vi "parseReadCalibrationResponse.vi"(8 "error in (no error)":errorcluster, 10 "DynamicFrameParser":refnum<class "DynamicFrameParser.lvclass">, 11 "ILC in":refnum<class "ILC.lvclass">) -> (0 "error out":errorcluster, 3 "ILC out":refnum<class "ILC.lvclass">)   [LabVIEW 2015, in "RTILC.lvlib" / "ILC.lvclass"]
uses:
  ILC.lvclass
  Common_RT_Modbus/DynamicFrameParser/DynamicFrameParser.lvclass
  Common_RT_Modbus/DataTypes/ExceptionCodes.ctl
  ILC.lvclass/ILC.ctl
  Common_RT_Modbus/RTModbus.lvlib
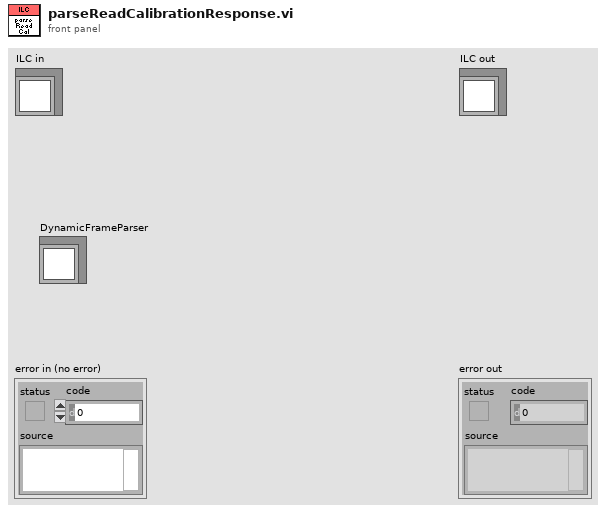
[diagram p1: front panel]
types:
  T1 = typedef "RTModbus.lvlib/ExceptionCodes.ctl" = u16
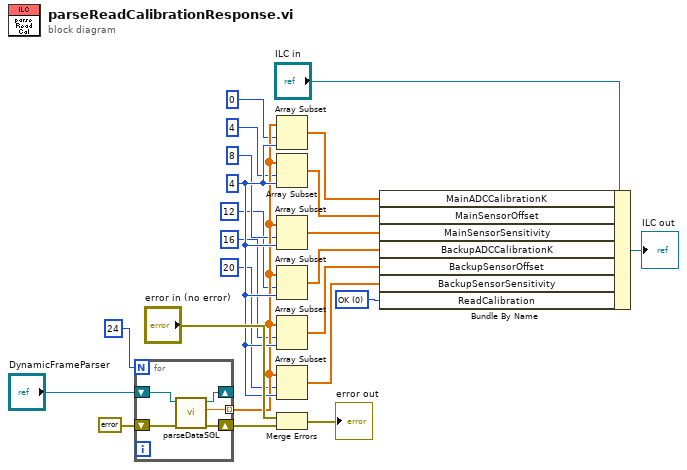
[diagram p0: block diagram]
diagram:
  w16 = 4
  w21 = T1 0 items=["OK", "IllegalFunction", "IllegalDataAddress", "IllegalDataValue", "SlaveDeviceFailure", "Acknowledge", "SlaveDeviceBusy", "NegativeAcknowledge", "MemoryParityError", "GatewayPathUnavailable", "GatewayTargetDeviceFailedToRespond"] ("ILCData.Responses.ILCMode")
  n1 = for {
    N: 24 -> [_]
    shift-right: [w27] -> _
    shift-left: "DynamicFrameParser" -> [w28]
    tunnel: [w26] -> w14 mode=indexing
    shift-right: [w25] -> w1
    shift-left: errorcluster {"status"=FALSE, "code"=0, "source"=""} ("error out") -> [w24]
    n2 = call "parseDataSGL.vi"("error in (no error)"=w24, "FrameParser in"=w28) -> ("error out"=w25:errorcluster, "Data"=w26:sgl, "FrameParser out"=w27:refnum<class "DynamicFrameParser.lvclass">)  [unwired: 7 in]
  }
  n3 = Array Subset(array=w14, index=0, length=w16) -> (w2:sgl[])
  n4 = Array Subset(array=w14, index=4, length=w16) -> (w3:sgl[])
  n5 = Array Subset(array=w14, index=8, length=w16) -> (w4:sgl[])
  n6 = Array Subset(array=w14, index=12, length=w16) -> (w5:sgl[])
  n7 = Array Subset(array=w14, index=16, length=w16) -> (w6:sgl[])
  n8 = Array Subset(array=w14, index=20, length=w16) -> (w7:sgl[])
  n9 = Merge Errors("error in (no error)", w1) -> (→"error out":errorcluster)
  n10 = Bundle By Name(cluster="ILC in", "MainADCCalibrationK"=w2, "MainSensorOffset"=w3, "MainSensorSensitivity"=w4, "BackupADCCalibrationK"=w5, "BackupSensorOffset"=w6, "BackupSensorSensitivity"=w7, "ReadCalibration"=w21) -> (→"ILC out":refnum<class "ILC.lvclass">)
